vi "灰度变换设置.vi"(8 "项目路径":path, 11 "图像输入":T1) -> (2 "是否应用":bool, 3 "图像":T1(plugin-control))   [LabVIEW 2018]
uses:
  <vilib>/vision/Image Controls.llb/IMAQ Image.ctl
  <vilib>/vision/NI_Vision_Development_Module.lvlib
panel:
  in  "多值分割":bool
  out "是否无ROI":bool
  out "遮罩":T1
  out "error out":errorcluster
  out "缓冲":T1(plugin-control)
  out "状态":T2
  in  "Lookup":bool
  in  "初始化":bool
  in  "应用":bool
  in  "二值化":bool
  in  "关闭":bool
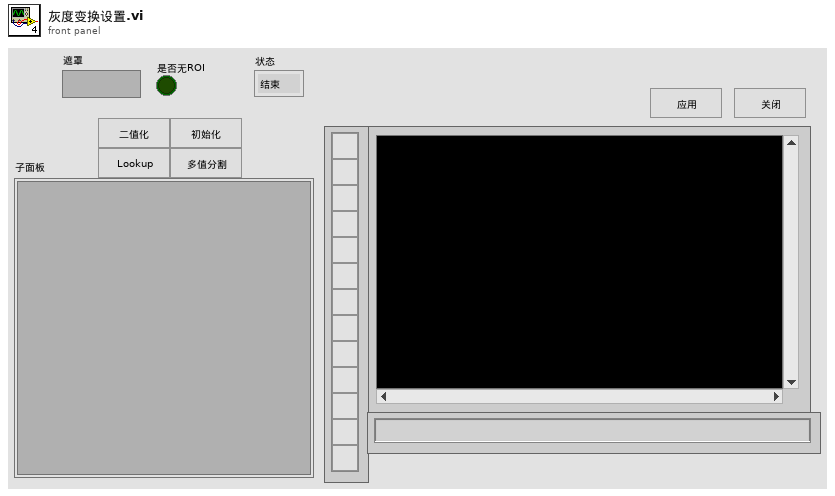
[diagram p1: front panel]
types:
  T1 = typedef "IMAQ Image.ctl" = refnum<image>
  T2 = typedef "状态机.ctl" = enum16{"结束", "运行1", "运行2", "运行3", "运行4", "运行5"}
  T3 = typedef "Image Type" = u32
  T4 = cluster{"Global Rectangle":i32[], "Contours":cluster{"Contour Type":u32, "ROI Type":u32, "Points":i32[]}[]}
  T5 = cluster{"Lower value":sgl, "Upper value":sgl, "Replace Value":sgl, "Keep/Replace Value (Replace)":bool}[]
  T6 = enum32{"Linear", "Log", "Exp", "Square", "Square root", "Power X", "Power 1/X"}
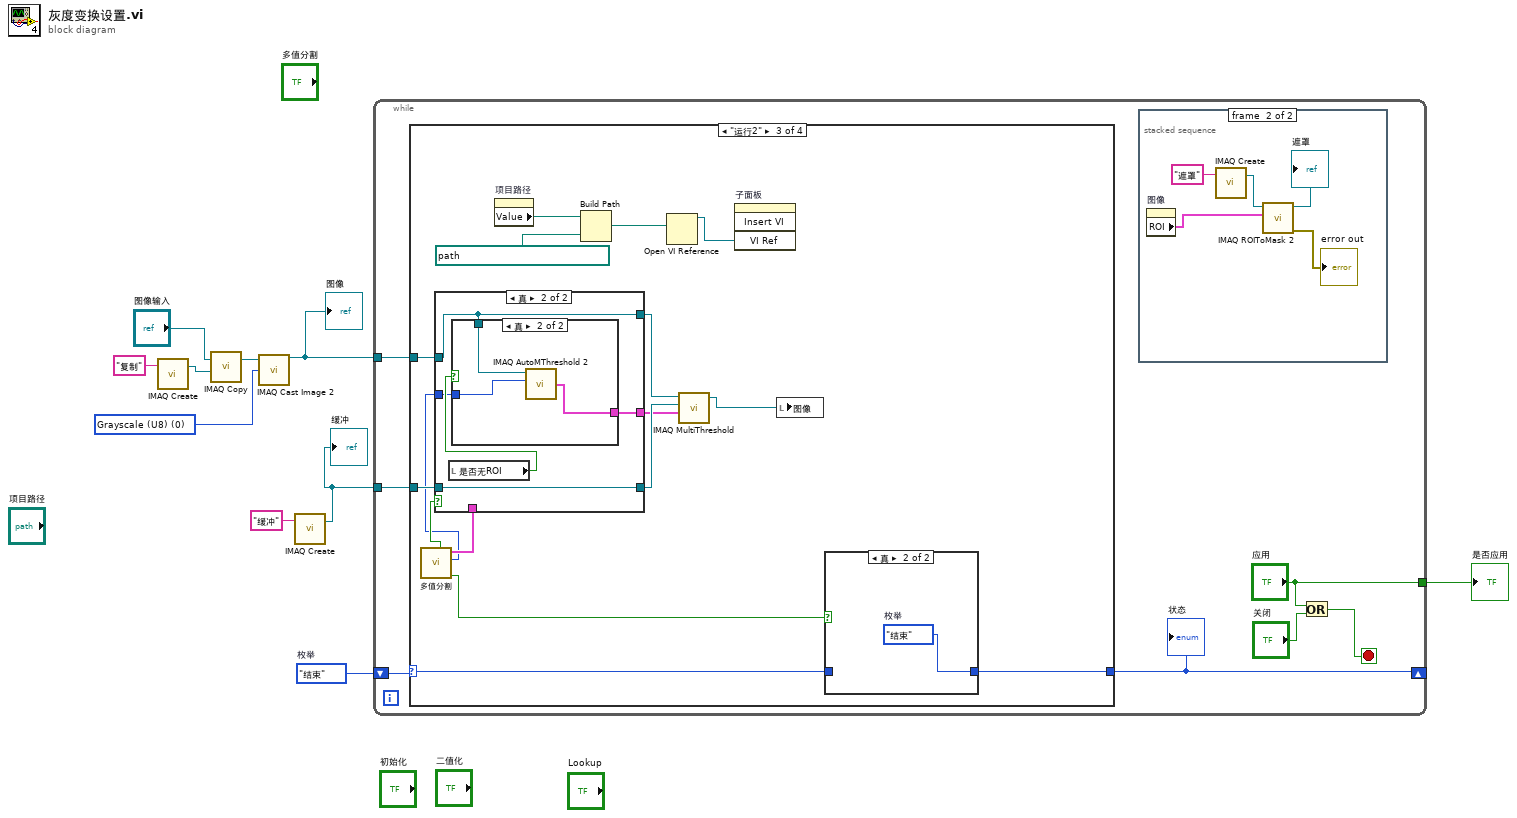
[diagram p0: block diagram]
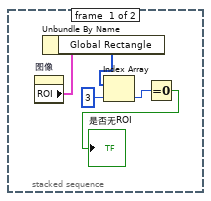
[diagram p2: hidden frame]
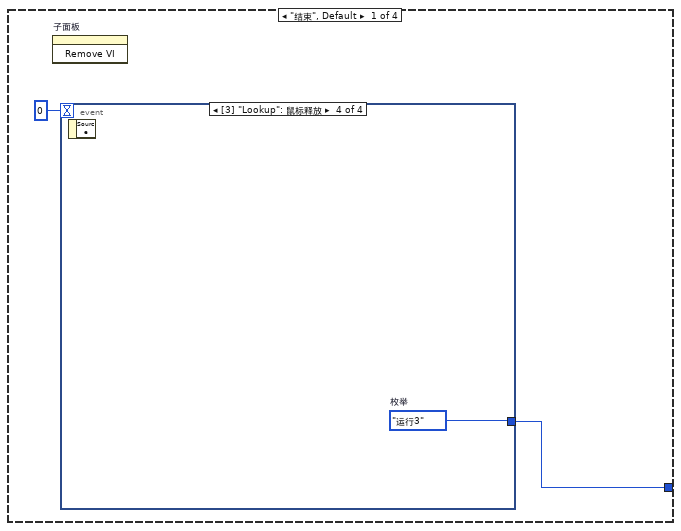
[diagram p3: hidden frame]
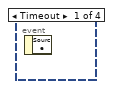
[diagram p4: hidden frame]
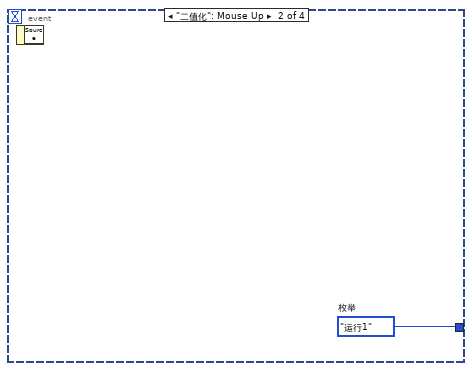
[diagram p5: hidden frame]
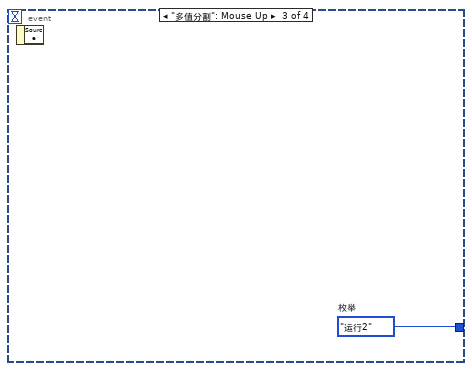
[diagram p6: hidden frame]
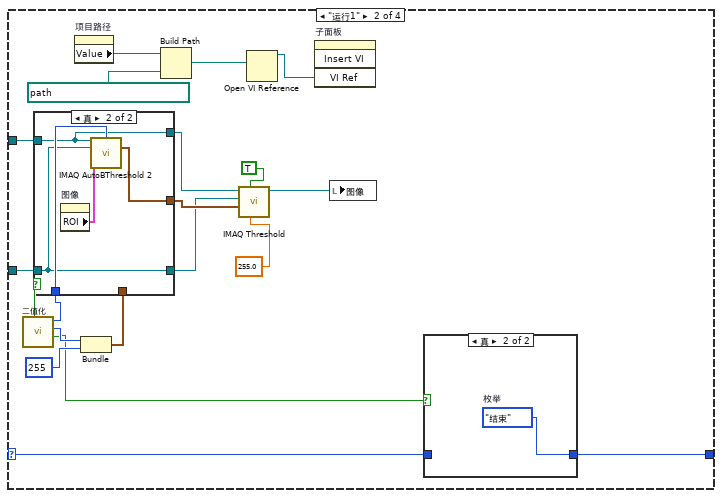
[diagram p7: hidden frame]
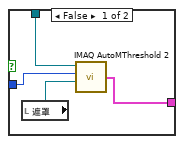
[diagram p11: hidden frame]
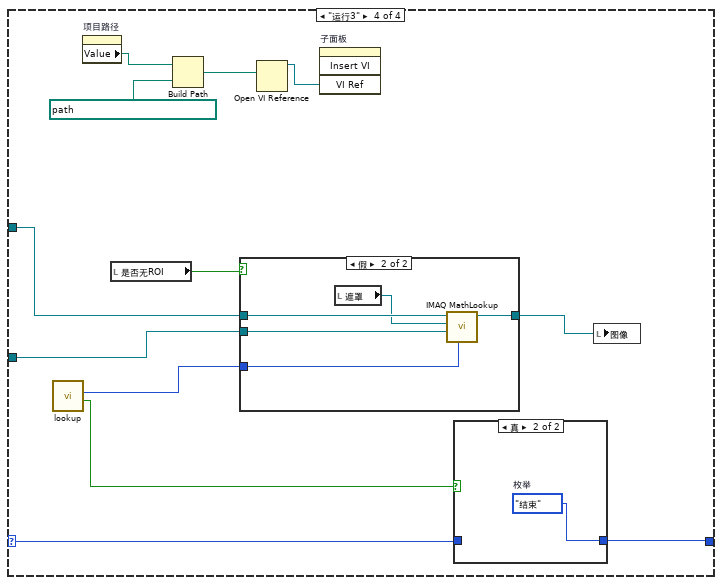
[diagram p13: hidden frame]
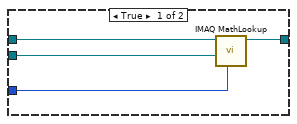
[diagram p15: hidden frame]
diagram:
  w3 = 状态机."结束"  # 枚举
  w6 = T3 0 items=["Grayscale (U8)", "Grayscale (I16)", "Grayscale (SGL)", "Complex (CSG)", "RGB (U32)", "HSL (U32)", "RGB (U64)", "Grayscale (U16)"] ("Image Type")
  n1 = call "IMAQ Create"("Image Name"="复制") -> ("New Image"=w8:T1)  [unwired: 4 in, 1 out]
  n2 = call "IMAQ Copy"("Image Dst"=w8, "Image Src"="图像输入") -> ("Image Dst Out"=w10:T1)  [unwired: 4 in, 1 out]
  n3 = call "IMAQ Cast Image 2"("Image Src"=w10, "Image Type"=w6) -> ("Image Dst Out"=w2:T1)  [unwired: 12 in, 1 out]
  "图像" <- w2
  n4 = call "IMAQ Create"("Image Name"="缓冲") -> ("New Image"=w1:T1)  [unwired: 4 in, 1 out]
  "缓冲" <- w1
  n5 = while {
    tunnel: ["应用"] -> w4
    shift-right: [w13] -> _
    shift-left: w3 -> [w14]
    tunnel: w2 -> [w12]
    tunnel: w1 -> [w11]
    stop <- w16 stop-if-true
    n6 = case shown="\"运行2\"" w14 {
      selector: w14 -> [_ w44 w76 w98]
      tunnel: [w29 w52 w78 w97] -> w13
      tunnel: w12 -> [_ w39 w72 w105]
      tunnel: w11 -> [_ w38 w71 w104]
      frame "结束", Default {
        n7 = invoke on="子面板" class="SubPnl" method="Remove VI"() -> ()  [unwired: 3 in, 3 out]
        n8 = event shown="[3] \"Lookup\": 鼠标释放" {
          selector: _ -> [_ _ _ _]
          dyn-events: _ -> [_ _ _ _]
          timeout: 0 -> [_ _ _ _]
          tunnel: [_ w30 w31 w32] -> w29
          event Timeout {
            n9 = event-data() -> ()  [unwired: 1 in, 1 out]
          }
          event "二值化": Mouse Up {
            w30 = 状态机."运行1"  # 枚举
            n10 = event-data() -> ()  [unwired: 1 in, 1 out]
          }
          event "多值分割": Mouse Up {
            w31 = 状态机."运行2"  # 枚举
            n11 = event-data() -> ()  [unwired: 1 in, 1 out]
          }
          event "Lookup": Mouse Up {
            w32 = 状态机."运行3"  # 枚举
            n12 = event-data() -> ()  [unwired: 1 in, 1 out]
          }
        }
      }
      frame "运行1" {
        n13 = call "二值化.vi"() -> ("确定"=w45:bool, "数值"=w50:u8, "方法"=w37:i32, "自动"=w40:bool)  [unwired: 6 in]
        n14 = property on="项目路径" class="Path"() -> ("Value"=w42:path)  [unwired: 2 in, 2 out]
        n15 = Bundle("数值"=w50, "Upper value"=u8 255) -> (w36:cluster{"数值":u8, "Upper value":u8})  [unwired: 1 in]
        n16 = case shown="真" w40 {
          tunnel: w39 -> [w54 w56]
          tunnel: w38 -> [w53 w57]
          tunnel: w37 -> [_ w59]
          tunnel: w36 -> [w55 _]
          tunnel: [w55 w58] -> w35
          tunnel: [w53 w57] -> w34
          tunnel: [w54 w56] -> w33
          frame False {
          }
          frame True {
            n17 = property on="图像" class="ImageControl"() -> ("ROI"=w60:T4)  [unwired: 2 in, 2 out]
            n18 = call "IMAQ AutoBThreshold 2"("Image Src"=w56, "Method (clustering)"=w59, "Image Dst"=w57, "ROI Descriptor"=w60) -> ("Threshold Range Out"=w58:cluster{"Lower value":sgl, "Upper value":sgl})  [unwired: 9 in, 2 out]
          }
        }
        n19 = Build Path(base path=w42, name or relative path=path "子vi/灰度变换子vi/二值化.vi" ("VI路径 2")) -> (appended path=w41:path)
        n20 = call "IMAQ Threshold"("Replace Value"=sgl 255.0, "Keep/Replace Value (Replace)"=TRUE, "Range"=w35, "Image Dst"=w34, "Image Src"=w33) -> ("Image Dst Out"=w46:T1)  [unwired: 5 in, 1 out]
        n21 = Open VI Reference(vi path=w41) -> (vi reference=w51:refnum<vi>)  [unwired: 5 in, 1 out]
        n22 = invoke on="子面板" class="SubPnl" method="Insert VI"("VI Ref"=w51) -> ()  [unwired: 3 in, 4 out]
        n23 = local write "图像"(w46) -> ()
        n24 = case shown="真" w45 {
          tunnel: [w61 w62] -> w52
          tunnel: w44 -> [w61 _]
          frame False {
          }
          frame True {
            w62 = 状态机."结束"  # 枚举
          }
        }
      }
      frame "运行2" {
        n25 = call "多值分割.vi"() -> ("确定"=w66:bool, "个数"=w63:u8, "阈值数组"=w64:T5, "自动"=w67:bool)  [unwired: 8 in]
        n26 = case shown="真" w67 {
          tunnel: w72 -> [w81 w84]
          tunnel: w71 -> [w80 w86]
          tunnel: [w80 w86] -> w69
          tunnel: [w81 w84] -> w70
          tunnel: [w79 w83] -> w65
          tunnel: w64 -> [w79 _]
          tunnel: w63 -> [_ w82]
          frame False {
          }
          frame True {
            n27 = local read "是否无ROI"() -> (w85:bool)
            n28 = case shown="真" w85 {
              tunnel: w84 -> [w90 w93]
              tunnel: [w89 w92] -> w83
              tunnel: w82 -> [w87 w91]
              frame False {
                n29 = local read "遮罩"() -> (w88:T1)
                n30 = call "IMAQ AutoMThreshold 2"("Image Mask"=w88, "Number of Classes"=w87, "Image"=w90) -> ("Threshold Data out"=w89:T5)  [unwired: 1 in, 2 out]
              }
              frame True {
                n31 = call "IMAQ AutoMThreshold 2"("Number of Classes"=w91, "Image"=w93) -> ("Threshold Data out"=w92:T5)  [unwired: 2 in, 2 out]
              }
            }
          }
        }
        n32 = property on="项目路径" class="Path"() -> ("Value"=w74:path)  [unwired: 2 in, 2 out]
        n33 = Build Path(base path=w74, name or relative path=path "子vi/灰度变换子vi/多值分割.vi" ("VI路径 2")) -> (appended path=w73:path)
        n34 = Open VI Reference(vi path=w73) -> (vi reference=w77:refnum<vi>)  [unwired: 5 in, 1 out]
        n35 = call "IMAQ MultiThreshold"("Threshold Data"=w65, "Image Dst"=w69, "Image Src"=w70) -> ("Image Dst Out"=w68:T1)  [unwired: 2 in, 1 out]
        n36 = invoke on="子面板" class="SubPnl" method="Insert VI"("VI Ref"=w77) -> ()  [unwired: 3 in, 4 out]
        n37 = local write "图像"(w68) -> ()
        n38 = case shown="真" w66 {
          tunnel: [w94 w95] -> w78
          tunnel: w76 -> [w94 _]
          frame False {
          }
          frame True {
            w95 = 状态机."结束"  # 枚举
          }
        }
      }
      frame "运行3" {
        n39 = call "lookup.vi"() -> ("确定"=w96:bool, "选择器 2"=w103:T6)  [unwired: 8 in]
        n40 = property on="项目路径" class="Path"() -> ("Value"=w100:path)  [unwired: 2 in, 2 out]
        n41 = local read "是否无ROI"() -> (w99:bool)
        n42 = Build Path(base path=w100, name or relative path=path "子vi/灰度变换子vi/lookup.vi" ("VI路径 3")) -> (appended path=w101:path)
        n43 = case shown="假" w99 {
          tunnel: [w113 w118] -> w106
          tunnel: w105 -> [w112 w117]
          tunnel: w104 -> [w111 w116]
          tunnel: w103 -> [w110 w115]
          frame True {
            n44 = call "IMAQ MathLookup"("Operator"=w110, "Image Dst"=w111, "Image Src"=w112) -> ("Image Dst Out"=w113:T1)  [unwired: 7 in, 1 out]
          }
          frame False {
            n45 = local read "遮罩"() -> (w114:T1)
            n46 = call "IMAQ MathLookup"("Operator"=w115, "Image Dst"=w116, "Image Mask"=w114, "Image Src"=w117) -> ("Image Dst Out"=w118:T1)  [unwired: 6 in, 1 out]
          }
        }
        n47 = Open VI Reference(vi path=w101) -> (vi reference=w107:refnum<vi>)  [unwired: 5 in, 1 out]
        n48 = invoke on="子面板" class="SubPnl" method="Insert VI"("VI Ref"=w107) -> ()  [unwired: 3 in, 4 out]
        n49 = case shown="真" w96 {
          tunnel: [w108 w109] -> w97
          tunnel: w98 -> [w108 _]
          frame False {
          }
          frame True {
            w109 = 状态机."结束"  # 枚举
          }
        }
        n50 = local write "图像"(w106) -> ()
      }
    }
    "状态" <- w13
    n51 = stacked-sequence {
      frame #0 {
        n52 = property on="图像" class="ImageControl"() -> ("ROI"=w20:T4)  [unwired: 2 in, 2 out]
        n53 = Unbundle By Name(w20) -> ("Global Rectangle"=w21:i32[])
        n54 = Index Array(array=w21, index=3 ("索引")) -> (element=w22:i32)
        n55 = Equal To 0?(x=w22) -> (x = 0?=→"是否无ROI":bool)
      }
      frame #1 {
        n56 = property on="图像" class="ImageControl"() -> ("ROI"=w25:T4)  [unwired: 2 in, 2 out]
        n57 = call "IMAQ Create"("Image Name"="遮罩") -> ("New Image"=w24:T1)  [unwired: 4 in, 1 out]
        n58 = call "IMAQ ROIToMask 2"("ROI Descriptor"=w25, "Image"=w24) -> ("error out"=→"error out":errorcluster, "Image Out"=→"遮罩":T1)  [unwired: 7 in, 1 out]
      }
    }
    n59 = Or(x="应用", y="关闭") -> (x .or. y?=w16:bool)
  }
  "是否应用" <- w4
